vi "Configure Delay.vi"(8 "error in (no error)":errorcluster, 10 "Delay (s)":dbl=0.001, 11 "VISA resource name":refnum<visa-resource-name>) -> (0 "error out":errorcluster, 3 "VISA resource name out":refnum<visa-resource-name>)   [LabVIEW 2020, in "QuPMXdriver.lvlib"]
doc: "Configures delay time that is required to prevent short circuit when the signal relays are opened and the ground relays are closed or viceversa. This time depends on the relays and load, but value should never decrease below 800 microseconds."
uses:
  QuPMXdriver.lvlib
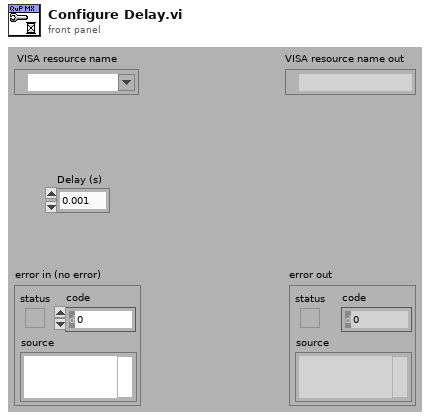
[diagram p1: front panel]
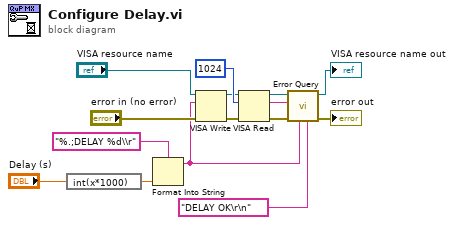
[diagram p0: block diagram]
diagram:
  n1 = expression code="int(x*1000)"("Delay (s)") -> (w3:dbl)
  n2 = Format Into String(format string="%.;DELAY %d\\r", w3) -> (resulting string=w4:string)  [unwired: 2 in, 1 out]
  n3 = VISA Write(VISA resource name="VISA resource name", write buffer=w4, error in (no error)="error in (no error)") -> (VISA resource name out=w7:refnum<visa-resource-name>, error out=w1:errorcluster)  [unwired: 1 out]
  n4 = VISA Read(VISA resource name=w7, byte count=u32 1024, error in (no error)=w1) -> (VISA resource name out=w8:refnum<visa-resource-name>, read buffer=w6:string, error out=w5:errorcluster)  [unwired: 1 out]
  n5 = call "Error Query.vi"("Expected read buffer"="DELAY OK\r\n" ("format string"), "Last command"=w4, "error in (no error)"=w5, "Read buffer"=w6, "VISA resource name"=w8) -> ("error out"=→"error out":errorcluster, "VISA resource name out"=→"VISA resource name out":refnum<visa-resource-name>)  [unwired: 5 in]
